vi "graph_prac.vi"() -> ()   [LabVIEW 2026]
panel:
  in  "stop":bool
  out "Waveform Chart":dbl(graph)
  out "Intensity Chart":dbl[][](graph)
  in  "Array":dbl[][](array[numeric])
  out "Intensity Graph":dbl[][](graph)
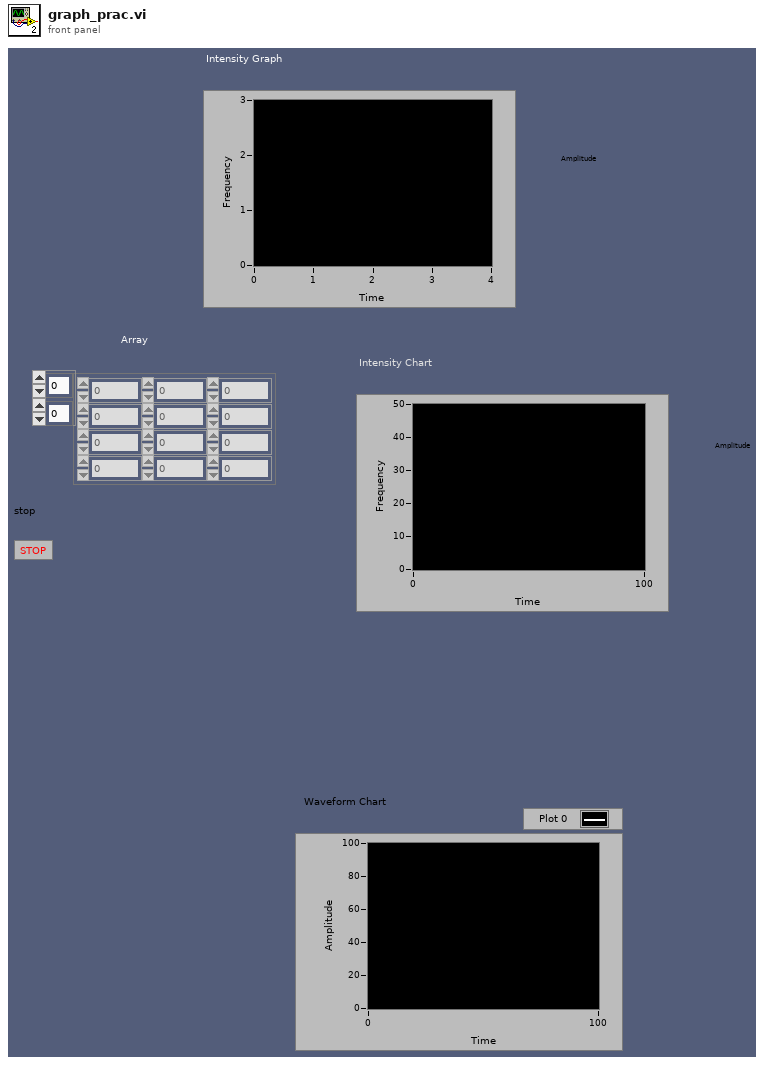
[diagram p1: front panel]
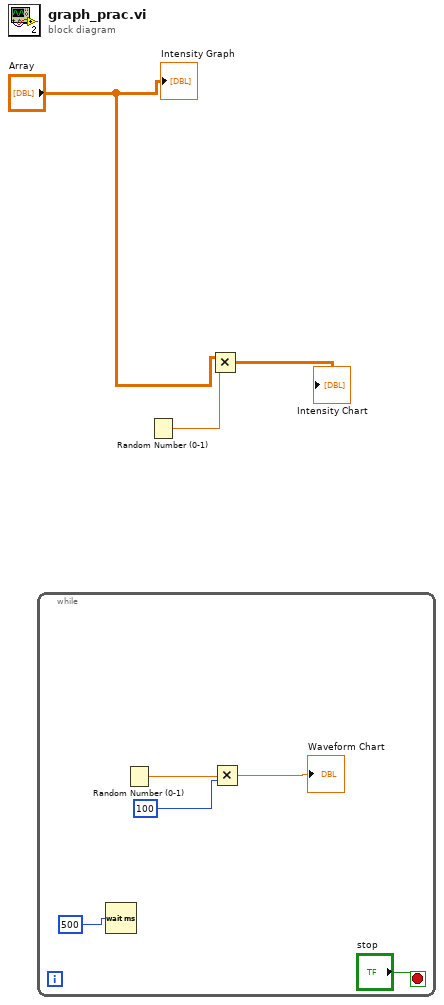
[diagram p0: block diagram]
diagram:
  n1 = while {
    stop <- "stop" stop-if-true
    n2 = Wait (ms)(milliseconds to wait=500) -> ()  [unwired: 1 out]
    n3 = Random Number (0-1)() -> (number: 0 to 1=w8:dbl)
    n4 = Multiply(x=w8, y=100) -> (x*y=→"Waveform Chart":dbl)
  }
  n5 = Random Number (0-1)() -> (number: 0 to 1=w1:dbl)
  n6 = Multiply(x="Array", y=w1) -> (x*y=→"Intensity Chart":dbl[][])
  "Intensity Graph" <- "Array"
